vi "Convert Timed Loop Time.vi"(11 "Actual Start [i]":i64) -> (3 "ET since start (s)":dbl)   [LabVIEW 2021, in "TCU Module.lvlib" / "TCU Module Engine.lvlib"]
uses:
  TCU Module Engine.lvlib
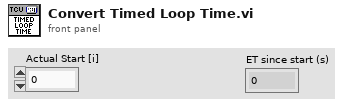
[diagram p1: front panel]
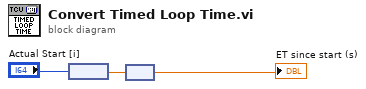
[diagram p0: block diagram]
diagram:
  n1 = node("Actual Start [i]") -> (w2:dbl[unit])
  n2 = node(w2) -> (→"ET since start (s)":dbl)
